vi "Flush Close Archive File.vi"(0 "TDMS File Refnum In":refnum<k34>, 5 "File Log Spec In":T1={"Directory"=path "", "Groups"=[], "Buffer Size"=0, "Properties"=[], "Pretrigger"=FALSE, "Pretrigger Samples"=0, "Name"="", "Timestamp"=FALSE, "Error"=0, "Auto Open"=FALSE, "File Node Ref"=0, "Archive"=FALSE, "Archive Directory"=path "", "Segment Files"=FALSE, "Segment Files By"=enum."Size", "Segment Size"=100000, "Flushed Data Size Total"=0, "Append Waveform Properties"=FALSE, "Logging State"=enum."Not Started", "First Sample Start Time"=timestamp(0 s since 1904-01-01), "System dt"=0.0} {"File Node Ref" format="%.0x"}, 11 "error in":errorcluster) -> (6 "File Log Spec Out":T1={"Directory"=path "", "Groups"=[], "Buffer Size"=0, "Properties"=[], "Pretrigger"=FALSE, "Pretrigger Samples"=0, "Name"="", "Timestamp"=FALSE, "Error"=0, "Auto Open"=FALSE, "File Node Ref"=0, "Archive"=FALSE, "Archive Directory"=path "", "Segment Files"=FALSE, "Segment Files By"=enum."Size", "Segment Size"=100000, "Flushed Data Size Total"=0, "Append Waveform Properties"=FALSE, "Logging State"=enum."Not Started", "First Sample Start Time"=timestamp(0 s since 1904-01-01), "System dt"=0.0} {"File Node Ref" format="%.0x"}, 15 "error out":errorcluster)   [LabVIEW 2027, in "Embedded Data Logger Engine.lvlib"]
uses:
  Embedded Data Logger Engine.lvlib
  File Logging Specification.ctl
  Group Logging Specification.ctl
  Group Buffer Data.ctl
  Property Specification.ctl
  <vilib>/NI VeriStand/Custom Device API/Custom Device Item Ref.ctl
  Shared/Segment Files By.ctl
  Logging State.ctl
  Flush Group Buffer.vi
  Add to Flushed Data Size.vi
  <vilib>/NI VeriStand/Custom Device API/Custom Device API.lvlib
  Shared/Embedded Data Logger Shared.lvlib
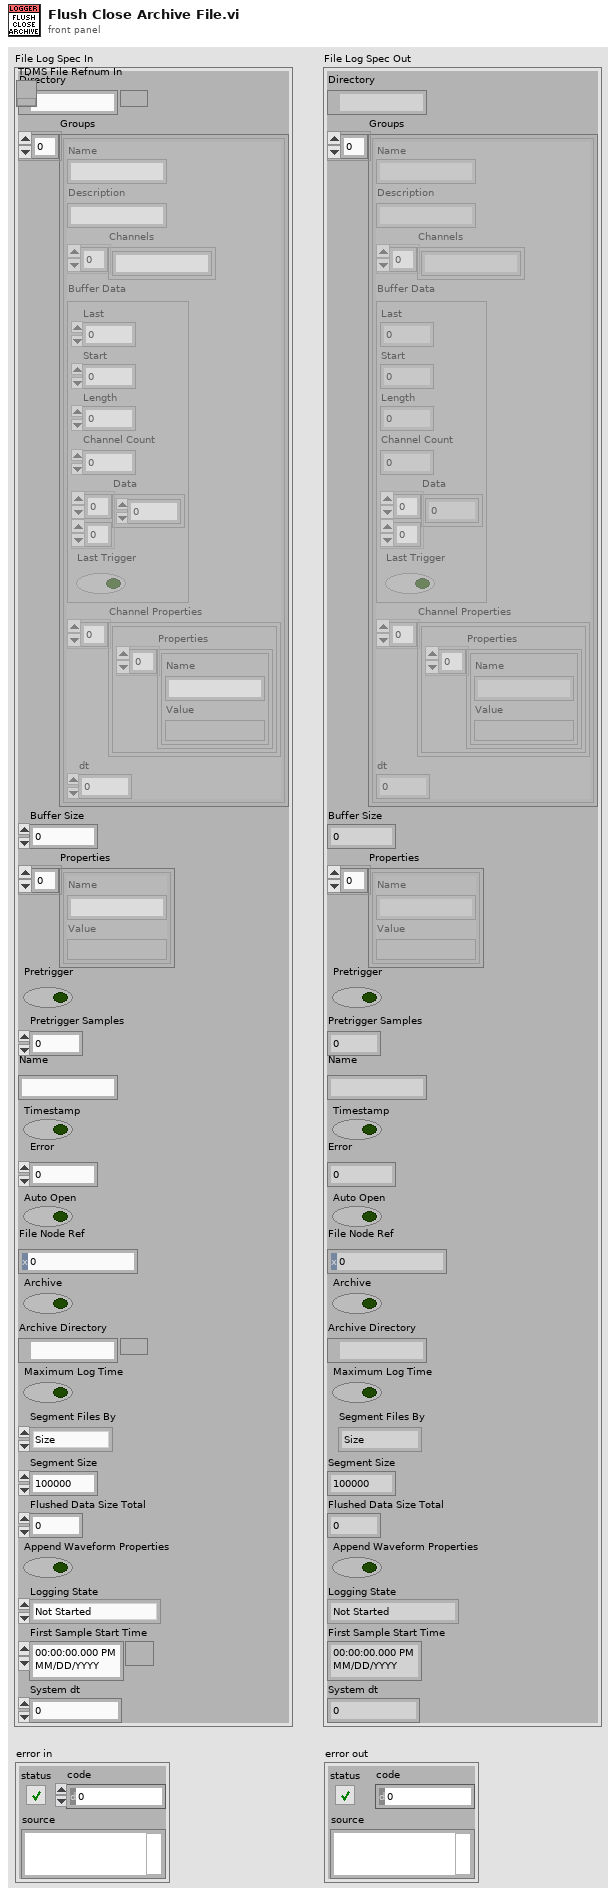
[diagram p1: front panel]
types:
  T1 = typedef "Embedded Data Logger Engine.lvlib/File Logging Specification.ctl" = cluster{"Directory":path, "Groups":T2[], "Buffer Size":i32, "Properties":T4[], "Pretrigger":bool, "Pretrigger Samples":i32, "Name":string, "Timestamp":bool, "Error":i32, "Auto Open":bool, "File Node Ref":T5, "Archive":bool, "Archive Directory":path, "Segment Files":bool, "Segment Files By":T6, "Segment Size":u32, "Flushed Data Size Total":u32, "Append Waveform Properties":bool, "Logging State":T7, "First Sample Start Time":timestamp, "System dt":dbl}
  T2 = typedef "Embedded Data Logger Engine.lvlib/Group Logging Specification.ctl" = cluster{"Name":string, "Description":string, "Channels":string[], "Buffer Data":T3, "Channel Properties":cluster{"Properties":T4[]}[], "dt":dbl}
  T3 = typedef "Embedded Data Logger Engine.lvlib/Group Buffer Data.ctl" = cluster{"Last":i32, "Start":i32, "Length":i32, "Channel Count":i32, "Data":dbl[][], "Last Trigger":bool}
  T4 = typedef "Embedded Data Logger Engine.lvlib/Property Specification.ctl" = cluster{"Name":string, "Value":variant}
  T5 = typedef "Custom Device API.lvlib/Custom Device Item Ref.ctl" = u64
  T6 = typedef "Embedded Data Logger Shared.lvlib/Segment Files By.ctl" = enum16{"Time", "Size"}
  T7 = typedef "Embedded Data Logger Engine.lvlib/Logging State.ctl" = enum16{"Not Started", "Continous Logging", "Paused", "Discontinous Logging"}
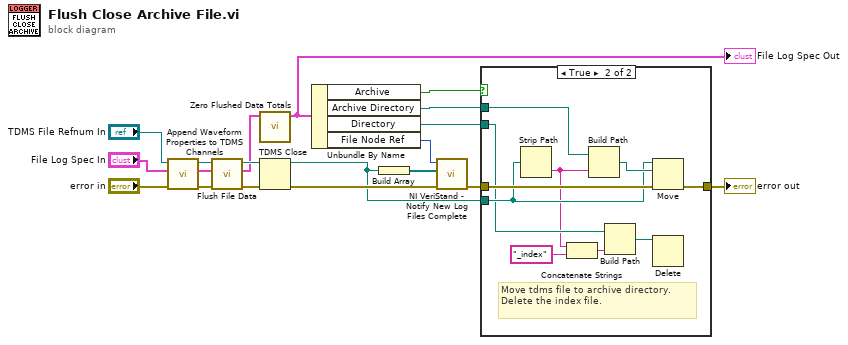
[diagram p0: block diagram]
diagram:
  n1 = call "Append Waveform Properties to TDMS Channels.vi"("error in"="error in", "File Log Spec In"="File Log Spec In", "TDMS File In"="TDMS File Refnum In") -> ("error out"=w5:errorcluster, "File Log Spec"=w1:T1, "TDMS File Out"=w3:refnum<k34>)  [unwired: 6 in]
  n2 = call "Flush File Data.vi"("error in (no error)"=w5, "File Log Spec in"=w1, "TDMS File Ref in"=w3) -> ("error out"=w17:errorcluster, "File Log Spec out"=w7:T1, "TDMS File Ref out"=w16:refnum<k34>)  [unwired: 6 in]
  n3 = call "Zero Flushed Data Totals.vi"("File Log Spec in"=w7) -> ("File Log Spec out"=w6:T1)  [unwired: 10 in]
  "File Log Spec Out" <- w6
  n4 = TDMS Close(8:w17, 11:w16) -> (0:w18:errorcluster, 3:w8:path)
  n5 = Unbundle By Name(w6) -> ("Archive"=w11:bool, "Archive Directory"=w14:path, "Directory"=w9:path, "File Node Ref"=w10:T5)
  n6 = Build Array(w8) -> (w19:path[])
  n7 = call <vilib>:"NI VeriStand - Notify New Log Files Complete.vi"("error in (no error)"=w18, "Log File Paths"=w19, "Item Ref in"=w10) -> ("error out"=w13:errorcluster)  [unwired: 6 in, 2 out]
  n8 = case shown="True" w11 {
    tunnel: w8 -> [_ w28]
    tunnel: w14 -> [_ w23]
    tunnel: w13 -> [w20 w29]
    tunnel: [w20 w22] -> w12
    tunnel: w9 -> [_ w24]
    frame False {
    }
    frame True {
      # "Move tdms file to archive directory. Delete the index file."
      n9 = Strip Path(path=w28) -> (name=w21:string)  [unwired: 1 out]
      n10 = Concatenate Strings(w21, "_index") -> (w27:string)
      n11 = Build Path(base path=w23, name or relative path=w21) -> (appended path=w30:path)
      n12 = Build Path(base path=w24, name or relative path=w27) -> (appended path=w26:path)
      n13 = Move(source path=w28, error in=w29, 10:w30) -> (error out=w22:errorcluster)  [unwired: 2 in, 2 out]
      n14 = Delete(path (use dialog)=w26) -> ()  [unwired: 4 in, 3 out]
    }
  }
  "error out" <- w12
